vi "ENED 1100 Task 3 9 29.vi"() -> ()   [LabVIEW 2016]
panel:
  out "Number of heads":dbl
  in  "Number of flips":dbl
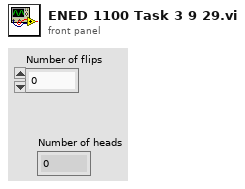
[diagram p1: front panel]
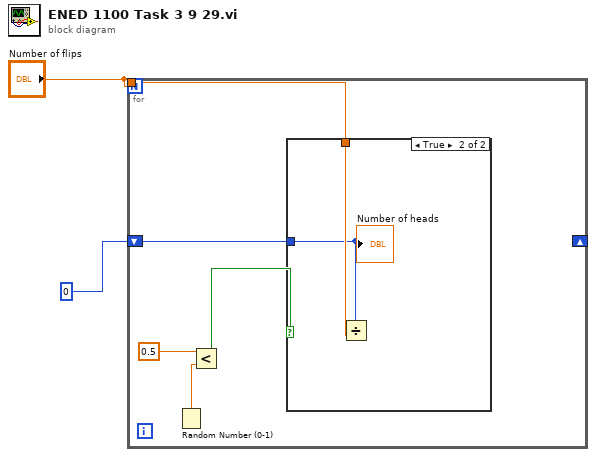
[diagram p0: block diagram]
diagram:
  n1 = for {
    N: "Number of flips" -> [_]
    shift-right: _ -> [_]
    shift-left: 0 -> [w4]
    tunnel: "Number of flips" -> [w3]
    n2 = Random Number (0-1)() -> (number: 0 to 1=w7:dbl)
    n3 = Less?(x=0.5, y=w7) -> (x < y?=w5:bool)
    n4 = case shown="True" w5 {
      tunnel: w4 -> [_ w8]
      tunnel: w3 -> [_ w9]
      frame False {
      }
      frame True {
        n5 = Divide(x=w8, y=w9) -> ()  [unwired: 1 out]
        "Number of heads" <- w8
      }
    }
  }
